vi "SwissSPAD Live_Select SS3 Gate Image.vi"(8 "Error In":errorcluster, 9 "Image to Display":T1, 10 "Gate 2 (500x250)":u8[][](array[numeric]), 11 "INT Gate (500x250)":u8[][](array[numeric])) -> (0 "Error Out":errorcluster, 3 "Selected Gate (500x250)":u8[][](array[numeric]), 4 "elapsed (relative) seconds":dbl)   [LabVIEW 2021]
uses:
  SwissSPAD Live_SS3 Displayed Image v2.ctl
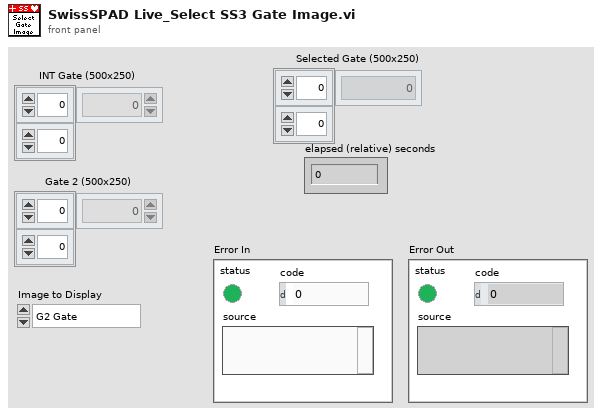
[diagram p1: front panel]
types:
  T1 = typedef "SwissSPAD Live_SS3 Displayed Image v2.ctl" = enum16{"G2 Gate", "INT Gate", "INT - G2"}
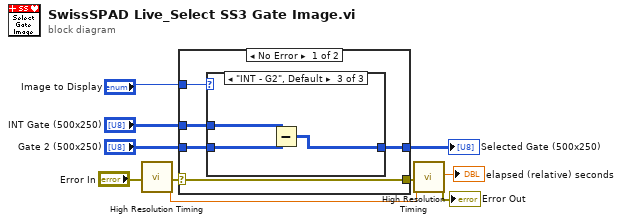
[diagram p0: block diagram]
diagram:
  n1 = call "High Resolution Timing.vi"("Error In"="Error In") -> ("elapsed (relative) seconds"=w2:dbl, "Error Out"=w4:errorcluster)  [unwired: 16 in, 1 out]
  n2 = case shown="No Error" w4 {
    selector: w4 -> [w11 w21]
    tunnel: "INT Gate (500x250)" -> [w15 _]
    tunnel: "Gate 2 (500x250)" -> [w14 _]
    tunnel: "Image to Display" -> [w13 _]
    tunnel: [w12 _] -> w7
    tunnel: [w11 w21] -> w5
    frame No Error {
      n3 = case shown="\"INT - G2\", Default" w13 {
        tunnel: [w16 w17 w20] -> w12
        tunnel: w14 -> [w16 _ w18]
        tunnel: w15 -> [_ w17 w19]
        frame "G2 Gate" {
        }
        frame "INT Gate" {
        }
        frame "INT - G2", Default {
          n4 = Subtract(x=w19, y=w18) -> (x-y=w20:u8[][])
        }
      }
    }
    frame Error {
    }
  }
  "Selected Gate (500x250)" <- w7
  n5 = call "High Resolution Timing.vi"("relative seconds (NaN)"=w2, "Error In"=w5) -> ("elapsed (relative) seconds"=→"elapsed (relative) seconds":dbl, "Error Out"=→"Error Out":errorcluster)  [unwired: 15 in, 1 out]
